vi "Live_Example_XCite_IMAQ.vi"() -> ()   [LabVIEW 2019]
doc: "This example demonstrates the image acquisition with one camera in ring buffer mode together with a live display of the latest images during record. Control of an X-Cite® light source is also possible. After record is stopped, the images can be addressed by index.\nNote that this example will not be fail save, i.e. doesnt react on errors, just handles them forward to the end\n\nUsage:\nSelect your required image count, data format and the camera setup before you start the program.\nOnce started, the camera class will be initialized and images will be recorded and displayed automatically\nYou can stop the images by pressing stop record.\nAfter stopped, the image at the selected index will be read out.\nA search for X-Cite® devices is started, and if found controls are initialized for each channel\nChannels can be switched on and off, and the intensity adjusted while the camera is acquiring images.\nWhen the recording is stopped, all the X-Cite® channels are switched off and controls are disabled.\nTo finish the program click on quit application, this will force an exit of the camera class\nYou can change your required ROI after and also during the record."
uses:
  camera/Camera.lvclass
  pco.sdk/TimingControl/TimingControl.lvlib
  <vilib>/Utility/miscctls.llb/LVOutOfRangeActionTypeDef.ctl
  xcite/Xcite.lvclass
panel:
  in  "type":u16(ring)=65535 items=["XC_120PC"=0, "XC_exacte"=1, "XC_120LED"=2, "XC_110LED"=3, "XC_mini"=4, "XC_XYLIS"=5, "XC_XR210"=6, "XC_LED1"=7, "XC_XT600"=8, "XC_XT900"=9, "Any"=65535]
  in  "Channel9_On":bool caption="735 nm"
  in  "Channel9_Intensity":u32 caption="735 nm" min=5 max=100
  in  "Channel8_On":bool caption="635 nm"
  in  "Channel8_Intensity":u32 caption="635 nm" min=5 max=100
  in  "Channel7_On":bool caption="580 nm"
  in  "Channel7_Intensity":u32 caption="580 nm" min=5 max=100
  in  "Channel6_On":bool caption="555 nm"
  in  "Channel6_Intensity":u32 caption="555 nm" min=5 max=100
  in  "Channel5_On":bool caption="510 nm"
  in  "Channel5_Intensity":u32 caption="510 nm" min=5 max=100
  in  "Channel4_On":bool caption="550 nm"
  in  "Channel4_Intensity":u32 caption="550 nm" min=5 max=100
  in  "Channel3_On":bool caption="475 nm"
  in  "Channel3_Intensity":u32 caption="475 nm" min=5 max=100
  in  "Channel2_On":bool caption="430 nm"
  in  "Channel2_Intensity":u32 caption="430 nm" min=5 max=100
  in  "Channel1_On":bool caption="385 nm"
  in  "Channel1_Intensity":u32 caption="385 nm" min=5 max=100
  out "X-Cite® Model":u16(ring)=65535 items=["XC_120PC"=0, "XC_exacte"=1, "XC_120LED"=2, "XC_110LED"=3, "XC_mini"=4, "XC_XYLIS"=5, "XC_XR210"=6, "XC_LED1"=7, "XC_XT600"=8, "XC_XT900"=9, "Any"=65535]
  in  "Trigger":bool
  in  "data_format":T1(ring)=enum."Mono16"
  out "Image":T2(plugin-control)
  out "rawImage":u16[][](array[numeric])
  in  "Image Index":u32 max=9
  out "Recorded Images":u32
  in  "TriggerMode":T3(ring)
  in  "Quit":bool
  out "Error":errorcluster {"code" format="%x"}
  in  "Stop Record":bool
  out "Recording On":bool
  in  "cropY1":u64=2 min=1 max=1040 step=1
  in  "cropX1":u64=2 min=1 max=1392 step=1
  in  "cropY0":u64=1 min=1 max=1039 step=1
  in  "cropX0":u64=1 min=1 max=1391 step=1
  out "Image Height":u64
  out "Image Width":u64
  in  "dwImgCount":u32=10 caption="Required Number of Images" max=2397
  in  "Exposure Time [s]":dbl=0.010000000000000002 min=1e-06 max=60.0 step=0.001
  # "This example demonstrates the image acquisition with one camera in ring buffer mode together with a live display of the latest images during record. Control of an X-Cite® light source is also possible. After record is stopped, the images can be addressed by index.\nNote that this example will not be fail save, i.e. doesnt react on errors, just handles them forward to the end\n\nUsage:\nSelect your required image count, data format and the camera setup before you start the program.\nOnce started, the camera class will be initialized and images will be recorded and displayed automatically\nYou can stop the images by pressing stop record.\nAfter stopped, the image at the selected index will be read out.\nA search for X-Cite® devices is started, and if found controls are initialized for each channel\nChannels can be switched on and off, and the intensity adjusted while the camera is acquiring images.\nWhen the recording is stopped, all the X-Cite® channels are switched off and controls are disabled.\nTo finish the program click on quit application, this will force an exit of the camera class\nYou can change the cropped region during or after recording."
  # "pco.labview"
  # "Camera Setup"
  # "X-Cite® controls"
  # "Recording Control"
  # "Parameters for image readout"
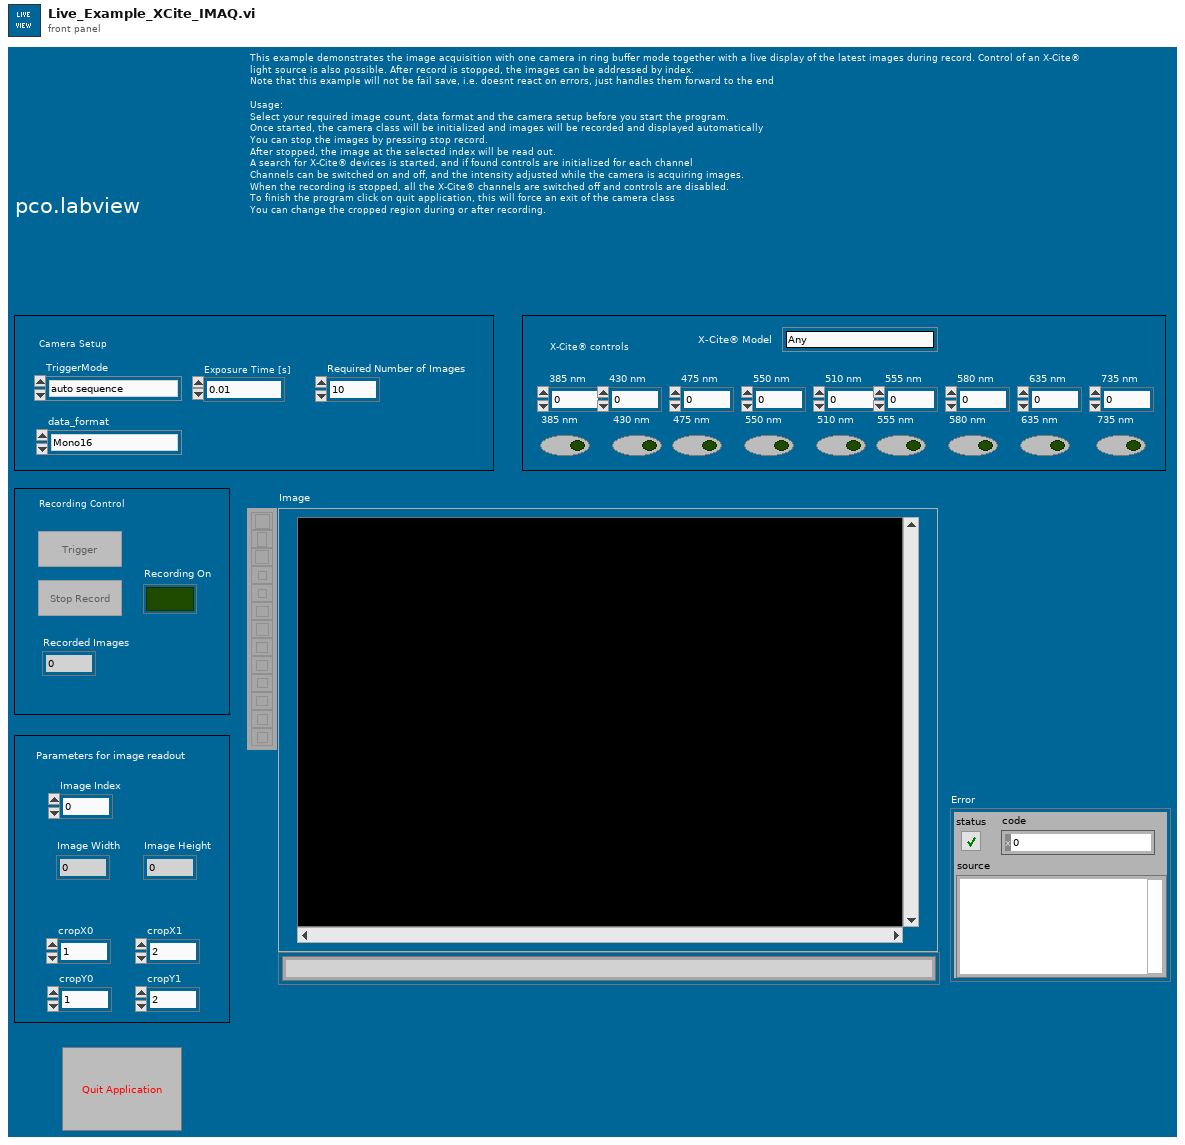
[diagram p1: front panel]
types:
  T1 = enum16{"Undefined", "Mono8", "Mono16", "BGRA8", "RGBA8", "BGRA16", "RGBA16", "CompressedMono8"}
  T2 = typedef "IMAQ Image.ctl" = refnum<image>
  T3 = enum16{"auto sequence", "software trigger", "external exposure start", "external exposure control"}
  T4 = enum8{"Enabled", "Disabled", "Disabled and Grayed Out"}
  T5 = cluster{"serial":u32, "type":u16, "name":string, "wavelenghts_vec":u32[], "exclusivity_vec":u32[], "intensity_max_vec":u32[], "intensity_min_vec":u32[]}
  T6 = enum16{"sequence", "sequence non blocking", "ring buffer", "fifo", "tif", "multitif", "pcoraw", "b16", "dicom", "multidicom", "camram_ring", "camram_segment"}
  T7 = typedef "LVOutOfRangeActionTypeDef.ctl" = cluster{"Out of Range Action Minimum":u8, "Out of Range Action Maximum":u8, "Out of Range Action Increment":u8}
  T8 = cluster{"serial":u32, "type":u16, "sub_type":u16, "interface_type":u16, "bit_resolution":u16, "min_exposure_time_s":dbl, "max_exposure_time_s":dbl, "min_exposure_step_s":dbl, "min_delay_time_s":dbl, "max_delay_time_s":dbl, "min_delay_step_s":dbl, "min_width":u64, "min_height":u64, "max_width":u64, "max_height":u64, "roi_step_horz":u64, "roi_step_vert":u64, "roi_symmetric_horz":bool, "roi_symmetric_vert":bool, "has_timestamp_mode":bool, "has_timestamp_mode_ascii_only":bool, "pixelrate_vec":u32[], "conversion_factor_vec":sgl[], "has_trigger_mode_extexpctrl":bool, "has_acquire_mode":bool, "has_ext_acquire_mode":bool, "has_metadata_mode":bool, "has_ram":bool, "binning_horz_vec":u16[], "binning_vert_vec":u16[], "has_average_binning":bool, "pixel_format_vec":u32[]}
  T9 = typedef "Image Type" = u32
  T10 = cluster{"wSignalNum":u16, "wEnabled":u16, "wType":u16, "wPolarity":u16, "wFilterSetting":u16, "wSelected":u16, "dwParameter":u32[], "dwSignalFunctionality":u32[]}
  T11 = typedef "Camera.lvclass/binning.ctl" = cluster{"vert":u16, "horz":u16, "mode":u16}
  T12 = cluster{"exposure_time_s":dbl, "delay_time_s":dbl, "roi":cluster{"x0":u64, "y0":u64, "x1":u64, "y1":u64}, "timestamp_mode":u16, "pixelrate":u32, "conversion_factor":sgl, "trigger_mode":u16, "acquire_mode":u16, "acquire_sequence_number":u32, "metadata_mode":u16, "noisefilter_mode":u16, "pixel_format":u32, "binning":T11, "auto_exposure":cluster{"region":u16, "min_exposure_s":dbl, "max_exposure_s":dbl}}
  T13 = cluster{"Plane 4 (alpha)":u16, "Plane 1 (Red)":u16, "Plane 2 (Green)":u16, "Plane 3 (Blue)":u16}[][]
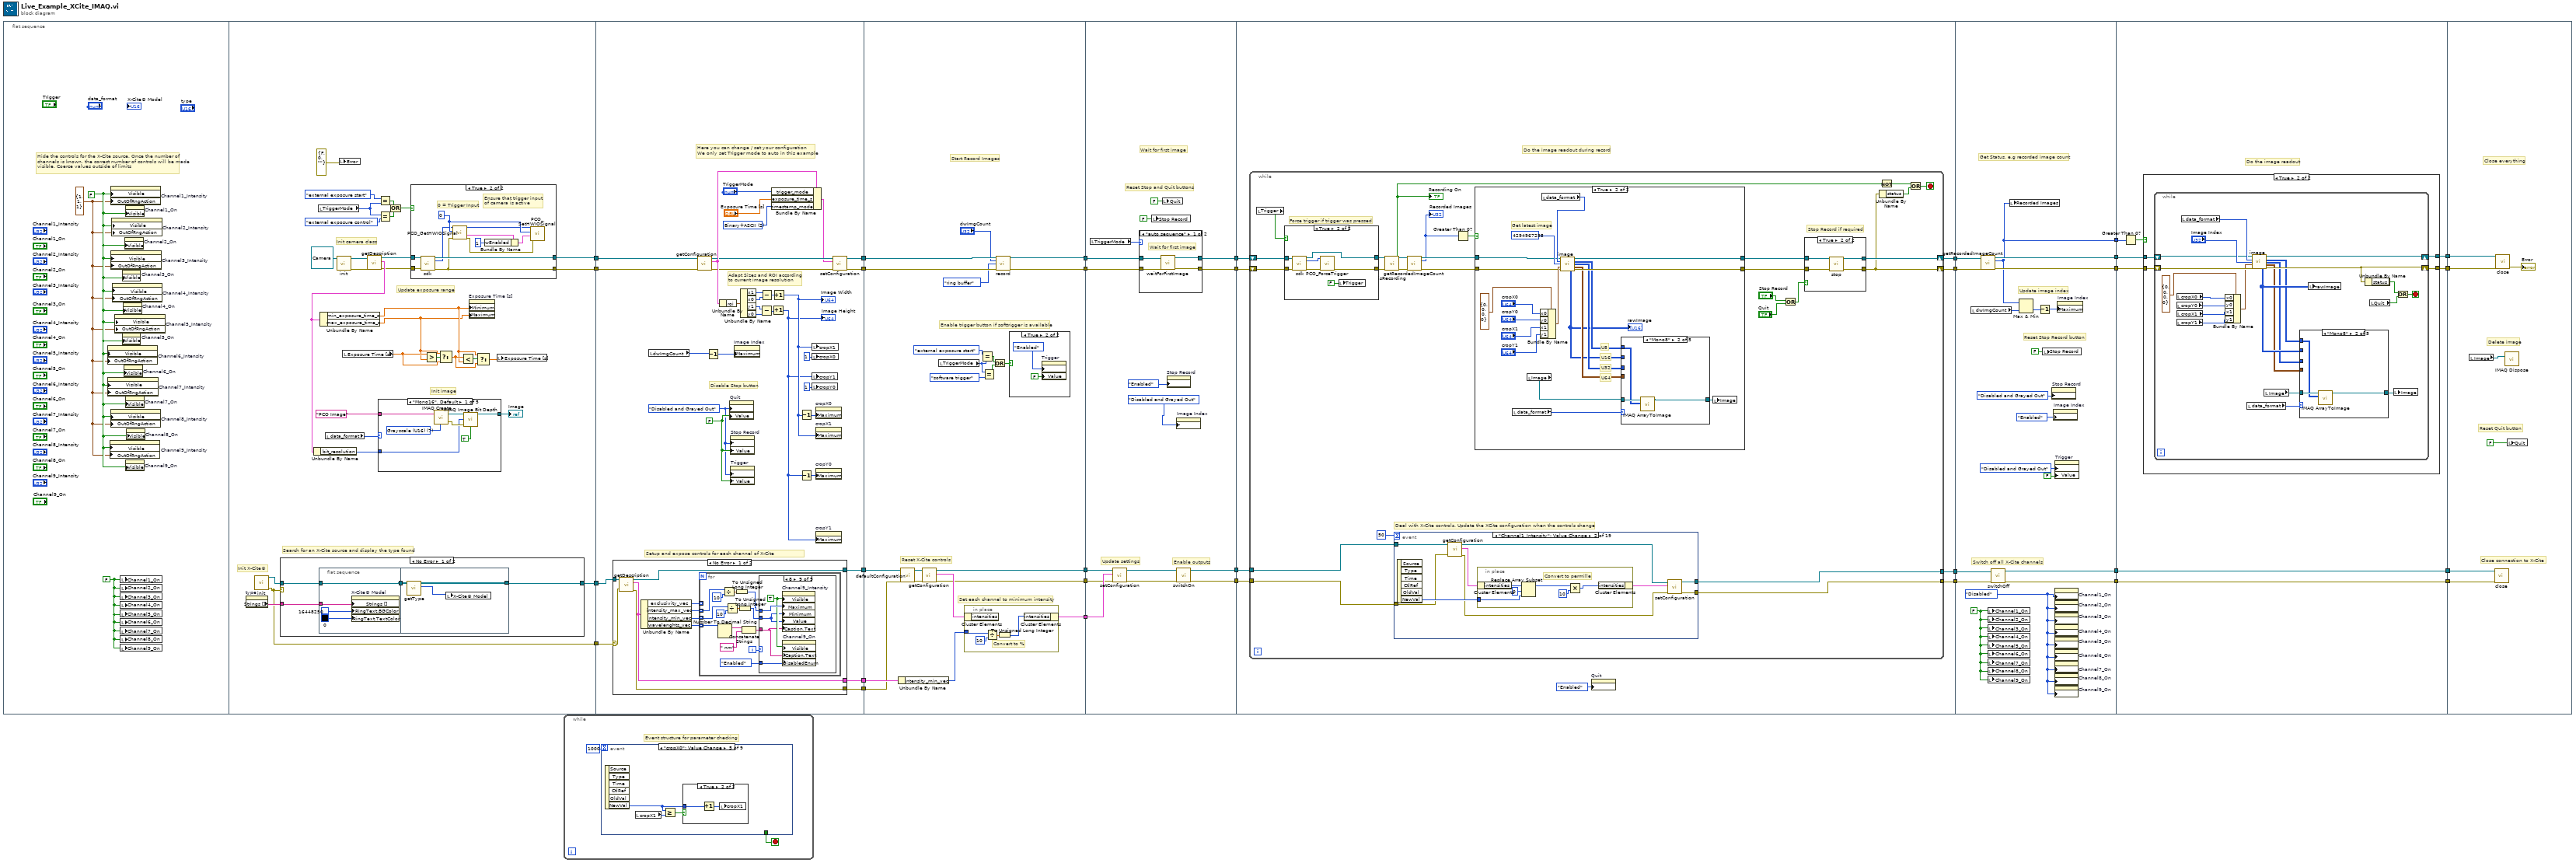
[diagram p0: block diagram]
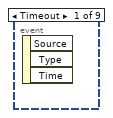
[diagram p2: hidden frame]
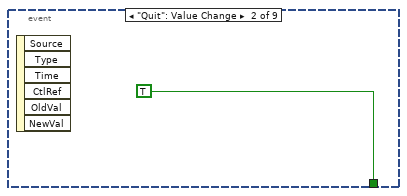
[diagram p3: hidden frame]
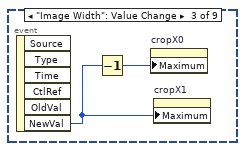
[diagram p4: hidden frame]
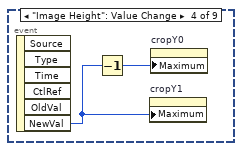
[diagram p5: hidden frame]
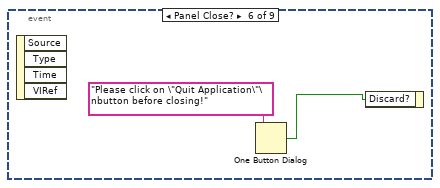
[diagram p7: hidden frame]
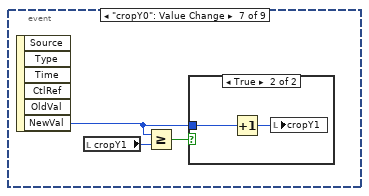
[diagram p8: hidden frame]
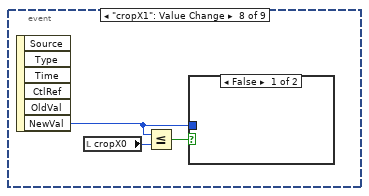
[diagram p10: hidden frame]
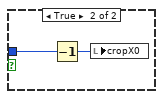
[diagram p11: hidden frame]
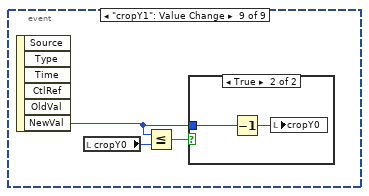
[diagram p12: hidden frame]
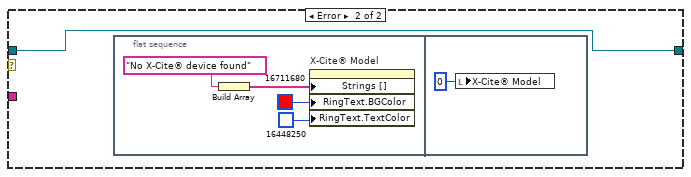
[diagram p14: hidden frame]
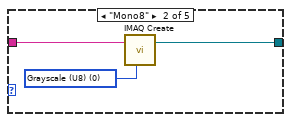
[diagram p16: hidden frame]
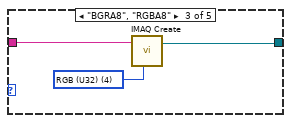
[diagram p17: hidden frame]
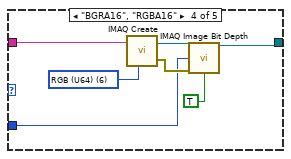
[diagram p18: hidden frame]
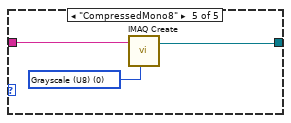
[diagram p19: hidden frame]
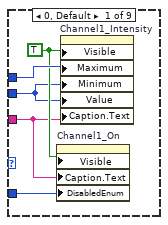
[diagram p20: hidden frame]
diagram:
  n1 = flat-sequence {
    tunnel: [w46] -> w23
    tunnel: [w45] -> w22
    tunnel: [w36] -> w16
    tunnel: [w35] -> w15
    tunnel: [w127] -> w31
    tunnel: [w131] -> w30
    tunnel: w23 -> [w126]
    tunnel: w22 -> [w125]
    tunnel: w16 -> [w122]
    tunnel: w15 -> [w121]
    tunnel: [w120] -> w14
    tunnel: [w119] -> w13
    tunnel: [w118] -> w12
    tunnel: [w233] -> w25
    tunnel: [w234] -> w24
    tunnel: w30 -> [w243]
    tunnel: w31 -> [w242]
    tunnel: w14 -> [w228]
    tunnel: w13 -> [w227]
    tunnel: w12 -> [w226]
    tunnel: [w225] -> w11
    tunnel: [w224] -> w10
    tunnel: [w223] -> w9
    tunnel: w25 -> [w261]
    tunnel: w24 -> [w262]
    tunnel: [w260] -> w29
    tunnel: [w258] -> w18
    tunnel: w11 -> [w254]
    tunnel: w10 -> [w250]
    tunnel: w9 -> [w253]
    tunnel: [w252] -> w8
    tunnel: [w251] -> w7
    tunnel: w29 -> [w280]
    tunnel: [w278] -> w28
    tunnel: [w277] -> w21
    tunnel: w18 -> [w276]
    tunnel: w8 -> [w275]
    tunnel: w7 -> [w274]
    tunnel: [w273] -> w6
    tunnel: [w272] -> w5
    tunnel: w28 -> [w637]
    tunnel: [w635] -> w27
    tunnel: w21 -> [w630]
    tunnel: [w629] -> w20
    tunnel: [w628] -> w17
    tunnel: w6 -> [w625]
    tunnel: w5 -> [w624]
    tunnel: [w623] -> w4
    tunnel: [w622] -> w3
    tunnel: w27 -> [w648]
    tunnel: [w647] -> w26
    tunnel: w20 -> [w646]
    tunnel: [w645] -> w19
    tunnel: w17 -> [w643]
    tunnel: w4 -> [w642]
    tunnel: w3 -> [w641]
    tunnel: [w642] -> w2
    tunnel: [w641] -> w1
    tunnel: w26 -> [w697]
    tunnel: w19 -> [w695]
    tunnel: w2 -> [w693]
    tunnel: w1 -> [w692]
    frame #0 {
      w32 = FALSE ("Channel1_On")
      w33 = T7 {"Out of Range Action Minimum"=1, "Out of Range Action Maximum"=1, "Out of Range Action Increment"=1} ("Response to Value Outside Limits")
      w34 = FALSE
      # "Hide the controls for the X-Cite source. Once the number of channels is known, the correct number of controls will be made visible. Coerce values outside of limits"
      n2 = property on="Channel6_Intensity" class="DigNum (strict)"("Visible"=w34, "OutOfRngAction"=w33) -> ()  [unwired: 2 in, 2 out]
      n3 = property on="Channel7_Intensity" class="DigNum (strict)"("Visible"=w34, "OutOfRngAction"=w33) -> ()  [unwired: 2 in, 2 out]
      n4 = property on="Channel9_Intensity" class="DigNum (strict)"("Visible"=w34, "OutOfRngAction"=w33) -> ()  [unwired: 2 in, 2 out]
      n5 = property on="Channel1_Intensity" class="DigNum (strict)"("Visible"=w34, "OutOfRngAction"=w33) -> ()  [unwired: 2 in, 2 out]
      n6 = property on="Channel8_Intensity" class="DigNum (strict)"("Visible"=w34, "OutOfRngAction"=w33) -> ()  [unwired: 2 in, 2 out]
      n7 = property on="Channel3_Intensity" class="DigNum (strict)"("Visible"=w34, "OutOfRngAction"=w33) -> ()  [unwired: 2 in, 2 out]
      n8 = property on="Channel2_Intensity" class="DigNum (strict)"("Visible"=w34, "OutOfRngAction"=w33) -> ()  [unwired: 2 in, 2 out]
      n9 = property on="Channel4_Intensity" class="DigNum (strict)"("Visible"=w34, "OutOfRngAction"=w33) -> ()  [unwired: 2 in, 2 out]
      n10 = property on="Channel5_Intensity" class="DigNum (strict)"("Visible"=w34, "OutOfRngAction"=w33) -> ()  [unwired: 2 in, 2 out]
      n11 = local write "Channel1_On"(w32) -> ()
      n12 = local write "Channel2_On"(w32) -> ()
      n13 = local write "Channel3_On"(w32) -> ()
      n14 = local write "Channel4_On"(w32) -> ()
      n15 = local write "Channel5_On"(w32) -> ()
      n16 = local write "Channel6_On"(w32) -> ()
      n17 = local write "Channel7_On"(w32) -> ()
      n18 = local write "Channel8_On"(w32) -> ()
      n19 = local write "Channel9_On"(w32) -> ()
      n20 = property on="Channel3_On" class="Bool (strict)"("Visible"=w34) -> ()  [unwired: 2 in, 2 out]
      n21 = property on="Channel5_On" class="Bool (strict)"("Visible"=w34) -> ()  [unwired: 2 in, 2 out]
      n22 = property on="Channel4_On" class="Bool (strict)"("Visible"=w34) -> ()  [unwired: 2 in, 2 out]
      n23 = property on="Channel6_On" class="Bool (strict)"("Visible"=w34) -> ()  [unwired: 2 in, 2 out]
      n24 = property on="Channel2_On" class="Bool (strict)"("Visible"=w34) -> ()  [unwired: 2 in, 2 out]
      n25 = property on="Channel7_On" class="Bool (strict)"("Visible"=w34) -> ()  [unwired: 2 in, 2 out]
      n26 = property on="Channel9_On" class="Bool (strict)"("Visible"=w34) -> ()  [unwired: 2 in, 2 out]
      n27 = property on="Channel1_On" class="Bool (strict)"("Visible"=w34) -> ()  [unwired: 2 in, 2 out]
      n28 = property on="Channel8_On" class="Bool (strict)"("Visible"=w34) -> ()  [unwired: 2 in, 2 out]
    }
    frame #1 {
      # "Search for an X-Cite source and display the type found"
      # "Init X-Cite®"
      # "Init image"
      # "Init camera class"
      # "Update exposure range"
      n29 = property on="type" class="Ring (strict)"() -> ("Strings []"=w37:string[])  [unwired: 2 in, 2 out]
      n30 = call "init.vi"() -> ("error out"=w35:errorcluster, "Xcite out"=w38:refnum<class "Xcite.lvclass">)  [unwired: 10 in]
      n31 = case shown="No Error" w35 {
        tunnel: w38 -> [w66 w76]
        tunnel: [w67 w76] -> w36
        tunnel: w37 -> [w68 _]
        frame No Error {
          n32 = flat-sequence {
            tunnel: w68 -> [w71]
            tunnel: w66 -> [w72]
            tunnel: [w72] -> w65
            tunnel: [w75] -> w67
            tunnel: w65 -> [w74]
            frame #0 {
              n33 = property on="X-Cite® Model" class="Ring (strict)"("Strings []"=w71, "RingText.BGColor"=u32 16448250 ("Ring Text.Colors:BG Color"), "RingText.TextColor"=u32 0 ("Ring Text.Colors:FG Color")) -> ()  [unwired: 2 in, 2 out]
            }
            frame #1 {
              n34 = call "getType.vi"("Xcite in"=w74) -> ("type"=w73:u16, "Xcite out"=w75:refnum<class "Xcite.lvclass">)  [unwired: 8 in, 1 out]
              n35 = local write "X-Cite® Model"(w73) -> ()
            }
          }
        }
        frame Error {
          n36 = flat-sequence {
            frame #0 {
              n37 = Build Array("No X-Cite® device found") -> (w79:string[])
              n38 = property on="X-Cite® Model" class="Ring (strict)"("Strings []"=w79, "RingText.BGColor"=u32 16711680 ("Ring Text.Colors:BG Color"), "RingText.TextColor"=u32 16448250 ("Ring Text.Text Colors:Text Color")) -> ()  [unwired: 2 in, 2 out]
            }
            frame #1 {
              n39 = local write "X-Cite® Model"(0) -> ()
            }
          }
        }
      }
      n40 = local read "TriggerMode"() -> (w40:T3)
      n41 = local read "data_format"() -> (w51:T1)
      n42 = call-dynamic "init.vi"("Camera in"=refnum<class "Camera.lvclass"> refnum) -> ("Camera out"=w54:refnum<class "Camera.lvclass">, "error out"=w55:errorcluster)  [unwired: 8 in]
      n43 = local write "Error"(errorcluster {"status"=FALSE, "code"=0, "source"=""} ("error IO")) -> ()
      n44 = local read "Exposure Time [s]"() -> (w63:dbl)
      n45 = call-dynamic "getDescription.vi"("error in (no error)"=w55, "Camera in"=w54) -> ("error out"=w47:errorcluster, "description"=w50:T8, "Camera out"=w48:refnum<class "Camera.lvclass">)  [unwired: 7 in]
      n46 = Unbundle By Name(w50) -> ("bit_resolution"=w49:u16)
      n47 = Unbundle By Name(w50) -> ("min_exposure_time_s"=w53:dbl, "max_exposure_time_s"=w52:dbl)
      n48 = case shown="\"Mono16\", Default" w51 {
        tunnel: "PCO Image" ("Image Name") -> [w100 w104 w106 w113 w116]
        tunnel: [w96 w102 w105 w110 w115] -> w56
        tunnel: w49 -> [w95 _ _ w108 _]
        frame "Mono16", Default {
          w101 = T9 7 items=["Grayscale (U8)", "Grayscale (I16)", "Grayscale (SGL)", "Complex (CSG)", "RGB (U32)", "HSL (U32)", "RGB (U64)", "Grayscale (U16)"] ("Image Type")
          n49 = call "IMAQ Create"("Image Name"=w100, "Image Type"=w101) -> ("New Image"=w98:T2, "error out"=w97:errorcluster)  [unwired: 3 in]
          n50 = call "IMAQ Image Bit Depth"("Image"=w98, "Bit Depth (0)"=w95, "error in (no error)"=w97, "Get/Set Bit Depth? (Set)"=TRUE) -> ("Image Out"=w96:T2)  [unwired: 9 in, 2 out]
        }
        frame "Mono8" {
          w103 = T9 0 items=["Grayscale (U8)", "Grayscale (I16)", "Grayscale (SGL)", "Complex (CSG)", "RGB (U32)", "HSL (U32)", "RGB (U64)", "Grayscale (U16)"] ("Image Type")
          n51 = call "IMAQ Create"("Image Name"=w104, "Image Type"=w103) -> ("New Image"=w102:T2)  [unwired: 3 in, 1 out]
        }
        frame "BGRA8", "RGBA8" {
          w107 = T9 4 items=["Grayscale (U8)", "Grayscale (I16)", "Grayscale (SGL)", "Complex (CSG)", "RGB (U32)", "HSL (U32)", "RGB (U64)", "Grayscale (U16)"] ("Image Type")
          n52 = call "IMAQ Create"("Image Name"=w106, "Image Type"=w107) -> ("New Image"=w105:T2)  [unwired: 3 in, 1 out]
        }
        frame "BGRA16", "RGBA16" {
          w114 = T9 6 items=["Grayscale (U8)", "Grayscale (I16)", "Grayscale (SGL)", "Complex (CSG)", "RGB (U32)", "HSL (U32)", "RGB (U64)", "Grayscale (U16)"] ("Image Type")
          n53 = call "IMAQ Create"("Image Name"=w113, "Image Type"=w114) -> ("New Image"=w111:T2, "error out"=w109:errorcluster)  [unwired: 3 in]
          n54 = call "IMAQ Image Bit Depth"("Image"=w111, "Bit Depth (0)"=w108, "error in (no error)"=w109, "Get/Set Bit Depth? (Set)"=TRUE) -> ("Image Out"=w110:T2)  [unwired: 9 in, 2 out]
        }
        frame "CompressedMono8" {
          w117 = T9 0 items=["Grayscale (U8)", "Grayscale (I16)", "Grayscale (SGL)", "Complex (CSG)", "RGB (U32)", "HSL (U32)", "RGB (U64)", "Grayscale (U16)"] ("Image Type")
          n55 = call "IMAQ Create"("Image Name"=w116, "Image Type"=w117) -> ("New Image"=w115:T2)  [unwired: 3 in, 1 out]
        }
      }
      "Image" <- w56
      n56 = Equal?(x=T3."external exposure start" ("TriggerMode"), y=w40) -> (x = y?=w43:bool)
      n57 = Equal?(x=w40, y=T3."external exposure control" ("TriggerMode")) -> (x = y?=w42:bool)
      n58 = Or(x=w43, y=w42) -> (x .or. y?=w41:bool)
      n59 = case shown="True" w41 {
        tunnel: w48 -> [w83 w88]
        tunnel: w47 -> [w82 w87]
        tunnel: [w83 w86] -> w46
        tunnel: [w82 w84] -> w45
        frame False {
        }
        frame True {
          w92 = u16 0 ("wSignalNum")
          # "0 = Trigger Input"
          # "Ensure that trigger input\nof camera is active"
          n60 = call-dynamic "sdk.vi"("Camera in"=w88, "error in (no error)"=w87) -> ("Camera out"=w86:refnum<class "Camera.lvclass">, "sdk"=w85:u64, "error out"=w84:errorcluster)  [unwired: 11 in]
          n61 = call "PCO_GetHWIOSignal.vi"("error in (no error)"=w84, "wSignalNum"=w92, "ph"=w85) -> ("error out"=w90:errorcluster, "strSignal"=w94:T10, "ph out"=w89:u64)  [unwired: 5 in, 1 out]
          n62 = Bundle By Name(cluster=w94, "wEnabled"=u16 1) -> (w91:T10)
          n63 = call "PCO_SetHWIOSignal.vi"("error in (no error)"=w90, "strSignal"=w91, "wSignalNum"=w92, "ph"=w89) -> ()  [unwired: 5 in, 3 out]
        }
      }
      n64 = Greater?(x=w63, y=w52) -> (0:w64:bool)
      n65 = Select(t=w52, s=w64, f=w63) -> (s? t:f=w61:dbl)
      n66 = Less?(x=w61, y=w53) -> (x < y?=w62:bool)
      n67 = property on="Exposure Time [s]" class="DigNum (strict)"("Minimum"=w53, "Maximum"=w52) -> ()  [unwired: 2 in, 2 out]
      n68 = Select(t=w53, s=w62, f=w61) -> (s? t:f=w60:dbl)
      n69 = local write "Exposure Time [s]"(w60) -> ()
    }
    frame #2 {
      w137 = u16 2 items=["OFF", "Binary", "Binary+ASCII", "ASCII"] ("wTimeStampMode")
      w124 = FALSE ("Stop")
      w123 = T4."Disabled and Grayed Out" ("Disabled")
      # "Setup and expose controls for each channel of X-Cite"
      # "Disable Stop button"
      # "Adapt Sizes and ROI according\nto current image resolution"
      # "Here you can change / set your configuration\nWe only set Trigger mode to auto in this example"
      n70 = case shown="No Error" w121 {
        selector: w121 -> [w152 w219]
        tunnel: w122 -> [w159 w221]
        tunnel: [w158 w221] -> w120
        tunnel: [w153 T5 {"serial"=0, "type"=0, "name"="", "wavelenghts_vec"=[], "exclusivity_vec"=[], "intensity_max_vec"=[], "intensity_min_vec"=[]} ("XCITE_Description")] -> w119
        tunnel: [w151 w219] -> w118
        frame No Error {
          n71 = call "getDescription.vi"("error in (no error)"=w152, "Xcite in"=w159) -> ("error out"=w151:errorcluster, "description"=w153:T5, "Xcite out"=w158:refnum<class "Xcite.lvclass">)  [unwired: 7 in]
          n72 = Unbundle By Name(w153) -> ("exclusivity_vec"=w157:u32[], "intensity_max_vec"=w156:u32[], "intensity_min_vec"=w155:u32[], "wavelenghts_vec"=w154:u32[])
          n73 = for {
            tunnel: w157 -> [_] mode=indexing
            tunnel: w156 -> [w167] mode=indexing
            tunnel: w155 -> [w162] mode=indexing
            tunnel: w154 -> [w172] mode=indexing
            i -> [w173]
            n74 = Number To Decimal String(number=w172) -> (decimal integer string=w171:string)  [unwired: 1 in]
            n75 = Divide(x=w167, y=u32 10) -> (x/y=w165:dbl)
            n76 = Divide(x=w162, y=u32 10) -> (x/y=w163:dbl)
            n77 = To Unsigned Long Integer(number=w165) -> (unsigned 32bit integer=w160:u32)
            n78 = To Unsigned Long Integer(number=w163) -> (unsigned 32bit integer=w161:u32)
            n79 = Concatenate Strings(w171, " nm") -> (w169:string)
            n80 = case shown="8" w173 {
              tunnel: w169 -> [w175 w180 w185 w191 w196 w201 w205 w211 w216]
              tunnel: w160 -> [w178 w183 w188 w193 w198 w203 w208 w213 w218]
              tunnel: w161 -> [w176 w181 w186 w190 w195 w200 w206 w210 w215]
              tunnel: T4."Enabled" ("Disabled") -> [w174 w179 w184 w189 w194 w199 w204 w209 w214]
              frame 0, Default {
                w177 = TRUE ("Visible")
                n81 = property on="Channel1_On" class="Bool (strict)"("Visible"=w177, "Caption.Text"=w175, "DisabledEnum"=w174) -> ()  [unwired: 2 in, 2 out]
                n82 = property on="Channel1_Intensity" class="DigNum (strict)"("Visible"=w177, "Maximum"=w178, "Minimum"=w176, "Value"=w176, "Caption.Text"=w175) -> ()  [unwired: 2 in, 2 out]
              }
              frame 1 {
                w182 = TRUE ("Visible")
                n83 = property on="Channel2_Intensity" class="DigNum (strict)"("Visible"=w182, "Maximum"=w183, "Minimum"=w181, "Value"=w181, "Caption.Text"=w180) -> ()  [unwired: 2 in, 2 out]
                n84 = property on="Channel2_On" class="Bool (strict)"("Visible"=w182, "Caption.Text"=w180, "DisabledEnum"=w179) -> ()  [unwired: 2 in, 2 out]
              }
              frame 2 {
                w187 = TRUE ("Visible")
                n85 = property on="Channel3_On" class="Bool (strict)"("Visible"=w187, "Caption.Text"=w185, "DisabledEnum"=w184) -> ()  [unwired: 2 in, 2 out]
                n86 = property on="Channel3_Intensity" class="DigNum (strict)"("Visible"=w187, "Maximum"=w188, "Minimum"=w186, "Value"=w186, "Caption.Text"=w185) -> ()  [unwired: 2 in, 2 out]
              }
              frame 3 {
                w192 = TRUE ("Visible")
                n87 = property on="Channel4_Intensity" class="DigNum (strict)"("Visible"=w192, "Maximum"=w193, "Minimum"=w190, "Value"=w190, "Caption.Text"=w191) -> ()  [unwired: 2 in, 2 out]
                n88 = property on="Channel4_On" class="Bool (strict)"("Visible"=w192, "Caption.Text"=w191, "DisabledEnum"=w189) -> ()  [unwired: 2 in, 2 out]
              }
              frame 4 {
                w197 = TRUE ("Visible")
                n89 = property on="Channel5_Intensity" class="DigNum (strict)"("Visible"=w197, "Maximum"=w198, "Minimum"=w195, "Value"=w195, "Caption.Text"=w196) -> ()  [unwired: 2 in, 2 out]
                n90 = property on="Channel5_On" class="Bool (strict)"("Visible"=w197, "Caption.Text"=w196, "DisabledEnum"=w194) -> ()  [unwired: 2 in, 2 out]
              }
              frame 5 {
                w202 = TRUE ("Visible")
                n91 = property on="Channel6_Intensity" class="DigNum (strict)"("Visible"=w202, "Maximum"=w203, "Minimum"=w200, "Value"=w200, "Caption.Text"=w201) -> ()  [unwired: 2 in, 2 out]
                n92 = property on="Channel6_On" class="Bool (strict)"("Visible"=w202, "Caption.Text"=w201, "DisabledEnum"=w199) -> ()  [unwired: 2 in, 2 out]
              }
              frame 6 {
                w207 = TRUE ("Visible")
                n93 = property on="Channel7_Intensity" class="DigNum (strict)"("Visible"=w207, "Maximum"=w208, "Minimum"=w206, "Value"=w206, "Caption.Text"=w205) -> ()  [unwired: 2 in, 2 out]
                n94 = property on="Channel7_On" class="Bool (strict)"("Visible"=w207, "Caption.Text"=w205, "DisabledEnum"=w204) -> ()  [unwired: 2 in, 2 out]
              }
              frame 7 {
                w212 = TRUE ("Visible")
                n95 = property on="Channel8_Intensity" class="DigNum (strict)"("Visible"=w212, "Maximum"=w213, "Minimum"=w210, "Value"=w210, "Caption.Text"=w211) -> ()  [unwired: 2 in, 2 out]
                n96 = property on="Channel8_On" class="Bool (strict)"("Visible"=w212, "Caption.Text"=w211, "DisabledEnum"=w209) -> ()  [unwired: 2 in, 2 out]
              }
              frame 8 {
                w217 = TRUE ("Visible")
                n97 = property on="Channel9_Intensity" class="DigNum (strict)"("Visible"=w217, "Maximum"=w218, "Minimum"=w215, "Value"=w215, "Caption.Text"=w216) -> ()  [unwired: 2 in, 2 out]
                n98 = property on="Channel9_On" class="Bool (strict)"("Visible"=w217, "Caption.Text"=w216, "DisabledEnum"=w214) -> ()  [unwired: 2 in, 2 out]
              }
            }
          }
        }
        frame Error {
        }
      }
      n99 = local read "dwImgCount"() -> (w138:u32)
      n100 = call-dynamic "getConfiguration.vi"("error in (no error)"=w125, "Camera in"=w126) -> ("error out"=w132:errorcluster, "configuration"=w143:T12, "Camera out"=w134:refnum<class "Camera.lvclass">)  [unwired: 7 in]
      n101 = Decrement(x=w138) -> (x-1=w128:u32)
      n102 = Unbundle By Name(w143) -> ("roi"=w144:cluster{"x0":u64, "y0":u64, "x1":u64, "y1":u64})
      n103 = property on="Quit" class="Bool (strict)"("DisabledEnum"=w123, "Value"=w124) -> ()  [unwired: 2 in, 2 out]
      n104 = property on="Stop Record" class="Bool (strict)"("DisabledEnum"=w123, "Value"=w124) -> ()  [unwired: 2 in, 2 out]
      n105 = property on="Trigger" class="Bool (strict)"("DisabledEnum"=w123, "Value"=w124) -> ()  [unwired: 2 in, 2 out]
      n106 = property on="Image Index" class="DigNum (strict)"("Maximum"=w128) -> ()  [unwired: 2 in, 2 out]
      n107 = Unbundle By Name(w144) -> ("x1"=w146:u64, "x0"=w145:u64, "y1"=w148:u64, "y0"=w147:u64)
      n108 = Subtract(x=w148, y=w147) -> (x-y=w150:u64)
      n109 = Subtract(x=w146, y=w145) -> (x-y=w149:u64)
      n110 = Bundle By Name(cluster=w143, "trigger_mode"="TriggerMode", "exposure_time_s"="Exposure Time [s]", "timestamp_mode"=w137) -> (w133:T12)
      n111 = Increment(x=w150) -> (x+1=w129:u64)
      "Image Height" <- w129
      n112 = Increment(x=w149) -> (x+1=w130:u64)
      "Image Width" <- w130
      n113 = Decrement(x=w130) -> (x-1=w141:u64)
      n114 = Decrement(x=w129) -> (x-1=w142:u64)
      n115 = local write "cropX1"(w130) -> ()
      n116 = local write "cropX0"(u64 1 ("roiY0")) -> ()
      n117 = local write "cropY1"(w129) -> ()
      n118 = local write "cropY0"(u64 1 ("roiY0")) -> ()
      n119 = property on="cropX0" class="DigNum (strict)"("Maximum"=w141) -> ()  [unwired: 2 in, 2 out]
      n120 = property on="cropX1" class="DigNum (strict)"("Maximum"=w130) -> ()  [unwired: 2 in, 2 out]
      n121 = property on="cropY0" class="DigNum (strict)"("Maximum"=w142) -> ()  [unwired: 2 in, 2 out]
      n122 = property on="cropY1" class="DigNum (strict)"("Maximum"=w129) -> ()  [unwired: 2 in, 2 out]
      n123 = call-dynamic "setConfiguration.vi"("error in (no error)"=w132, "configuration"=w133, "Camera in"=w134) -> ("error out"=w131:errorcluster, "Camera out"=w127:refnum<class "Camera.lvclass">)  [unwired: 7 in]
    }
    frame #3 {
      # "Set each channel to minimum intensity"
      # "Reset X-Cite controls"
      # "Enable trigger button if softtrigger is available"
      # "Start Record Images"
      n124 = Unbundle By Name(w227) -> ("intensity_min_vec"=w229:u32[])
      n125 = call "defaultConfiguration.vi"("error in (no error)"=w226, "Xcite in"=w228) -> ("error out"=w231:errorcluster, "Xcite out"=w232:refnum<class "Xcite.lvclass">)  [unwired: 8 in]
      n126 = call "getConfiguration.vi"("error in (no error)"=w231, "Xcite in"=w232) -> ("error out"=w224:errorcluster, "configuration"=w230:cluster{"intensities":u32[], "on_states":u8[]}, "Xcite out"=w225:refnum<class "Xcite.lvclass">)  [unwired: 7 in]
      n127 = local read "TriggerMode"() -> (w239:T3)
      n128 = in-place {
        in-place-border: w229 -> [w245]
        # "Convert to %"
        n129 = in-place-cluster #1(w230) -> ()  [unwired: 1 out]
        n130 = Divide(x=w245, y=u32 10) -> (x/y=w246:dbl[])
        n131 = To Unsigned Long Integer(number=w246) -> (unsigned 32bit integer=w244:u32[])
        n132 = in-place-cluster #1("intensities"=w244) -> (w223:cluster{"intensities":u32[], "on_states":u8[]})
      }
      n133 = Equal?(x=T3."external exposure start" ("TriggerMode"), y=w239) -> (x = y?=w236:bool)
      n134 = Equal?(x=w239, y=T3."software trigger" ("TriggerMode")) -> (x = y?=w235:bool)
      n135 = Or(x=w236, y=w235) -> (x .or. y?=w237:bool)
      n136 = call-dynamic "record.vi"("Camera in"=w242, "num_images"="dwImgCount", "record_mode"=T6."ring buffer", "error in (no error)"=w243) -> ("Camera out"=w234:refnum<class "Camera.lvclass">, "error out"=w233:errorcluster)  [unwired: 10 in]
      n137 = case shown="True" w237 {
        frame False {
        }
        frame True {
          n138 = property on="Trigger" class="Bool (strict)"("DisabledEnum"=T4."Enabled" ("Disabled"), "Value"=FALSE ("Trigger")) -> ()  [unwired: 2 in, 2 out]
        }
      }
    }
    frame #4 {
      # "Enable outputs"
      # "Update settings"
      # "Wait for first image"
      # "Reset Stop and Quit buttons"
      n139 = local read "TriggerMode"() -> (w257:T3)
      n140 = call "setConfiguration.vi"("error in (no error)"=w250, "configuration"=w253, "Xcite in"=w254) -> ("error out"=w255:errorcluster, "Xcite out"=w256:refnum<class "Xcite.lvclass">)  [unwired: 7 in]
      n141 = case shown="\"auto sequence\"" w257 {
        tunnel: w262 -> [w269 w271]
        tunnel: w261 -> [w268 w270]
        tunnel: [w267 w270] -> w260
        tunnel: [w266 w271] -> w258
        frame "auto sequence" {
          # "Wait for first image"
          n142 = call-dynamic "waitForFirstImage.vi"("error in (no error)"=w268, "Camera in"=w269) -> ("error out"=w267:errorcluster, "Camera out"=w266:refnum<class "Camera.lvclass">)  [unwired: 8 in]
        }
        frame Default {
        }
      }
      n143 = local write "Stop Record"(FALSE ("Stop Record")) -> ()
      n144 = local write "Quit"(FALSE ("Stop")) -> ()
      n145 = property on="Stop Record" class="Bool (strict)"("DisabledEnum"=T4."Enabled" ("Disabled")) -> ()  [unwired: 2 in, 2 out]
      n146 = property on="Image Index" class="DigNum (strict)"("DisabledEnum"=T4."Disabled and Grayed Out" ("Disabled")) -> ()  [unwired: 2 in, 2 out]
      n147 = call "switchOn.vi"("error in (no error)"=w255, "Xcite in"=w256) -> ("error out"=w251:errorcluster, "Xcite out"=w252:refnum<class "Xcite.lvclass">)  [unwired: 8 in]
    }
    frame #5 {
      # "Do the image readout during record"
      n148 = while {
        shift-right: [w288] -> w278
        shift-left: w280 -> [w292]
        shift-right: [w289] -> w277
        shift-left: w276 -> [w293]
        tunnel: w275 -> [w284]
        tunnel: w274 -> [w283]
        tunnel: [w282] -> w273
        tunnel: [w281] -> w272
        stop <- w304 stop-if-true
        # "Deal with X-Cite controls. Update the XCite configuration when the controls change"
        # "Force trigger if trigger was pressed"
        # "Stop Record if required"
        n149 = local read "Trigger"() -> (w294:bool)
        n150 = case shown="True" w294 {
          tunnel: w293 -> [w608 w613]
          tunnel: w292 -> [w607 w612]
          tunnel: [w608 w611] -> w291
          tunnel: [w607 w610] -> w290
          frame False {
          }
          frame True {
            n151 = call-dynamic "sdk.vi"("Camera in"=w613, "error in (no error)"=w612) -> ("Camera out"=w611:refnum<class "Camera.lvclass">, "sdk"=w614:u64, "error out"=w615:errorcluster)  [unwired: 11 in]
            n152 = call "PCO_ForceTrigger.vi"("error in (no error)"=w615, "ph"=w614) -> ("error out"=w610:errorcluster)  [unwired: 6 in, 3 out]
            n153 = local write "Trigger"(FALSE ("Trigger")) -> ()
          }
        }
        n154 = call-dynamic "isRecording.vi"("Camera in"=w291, "error in (no error)"=w290) -> ("Camera out"=w299:refnum<class "Camera.lvclass">, "recording"=w302:bool, "error out"=w298:errorcluster)  [unwired: 11 in]
        "Recording On" <- w302
        n155 = event shown="[1] \"Channel1_Intensity\": Value Change" {
          selector: _ -> [_ _ _ _ _ _ _ _ _ _ _ _ _ _ _ _ _ _ _]
          dyn-events: _ -> [_ _ _ _ _ _ _ _ _ _ _ _ _ _ _ _ _ _ _]
          timeout: 50 -> [_ _ _ _ _ _ _ _ _ _ _ _ _ _ _ _ _ _ _]
          tunnel: w284 -> [w308 w316 w331 w346 w361 w376 w391 w406 w421 w436 w452 w466 w480 w494 w508 w522 w536 w550 w564]
          tunnel: [w309 w315 w330 w345 w360 w375 w390 w405 w420 w435 w451 w465 w479 w493 w507 w521 w535 w549 w563] -> w281
          tunnel: w283 -> [w309 w311 w326 w341 w356 w371 w386 w401 w416 w431 w446 w460 w474 w488 w502 w516 w530 w544 w558]
          tunnel: [w308 w314 w329 w344 w359 w374 w389 w404 w419 w434 w450 w464 w478 w492 w506 w520 w534 w548 w562] -> w282
          event Timeout {
            n156 = event-data() -> ()  [unwired: 1 in, 3 out]
          }
          event "Channel1_Intensity": Value Change {
            n157 = event-data() -> ("NewVal"=w318:u32)  [unwired: 1 in, 5 out]
            n158 = call "getConfiguration.vi"("error in (no error)"=w311, "Xcite in"=w316) -> ("error out"=w310:errorcluster, "configuration"=w312:cluster{"intensities":u32[], "on_states":u8[]}, "Xcite out"=w313:refnum<class "Xcite.lvclass">)  [unwired: 7 in]
            n159 = in-place {
              in-place-border: w318 -> [w322]
              # "Convert to permille"
              n160 = in-place-cluster #2(w312) -> ("intensities"=w324:u32[])
              n161 = Replace Array Subset(array=w324, new element=w322, index=0) -> (w320:u32[])
              n162 = Multiply(x=w320, y=u32 10) -> (x*y=w319:u32[])
              n163 = in-place-cluster #2("intensities"=w319) -> (w317:cluster{"intensities":u32[], "on_states":u8[]})
            }
            n164 = call "setConfiguration.vi"("error in (no error)"=w310, "configuration"=w317, "Xcite in"=w313) -> ("error out"=w315:errorcluster, "Xcite out"=w314:refnum<class "Xcite.lvclass">)  [unwired: 7 in]
          }
          event "Channel2_Intensity": Value Change {
            n165 = event-data() -> ("NewVal"=w333:u32)  [unwired: 1 in, 5 out]
            n166 = call "getConfiguration.vi"("error in (no error)"=w326, "Xcite in"=w331) -> ("error out"=w325:errorcluster, "configuration"=w327:cluster{"intensities":u32[], "on_states":u8[]}, "Xcite out"=w328:refnum<class "Xcite.lvclass">)  [unwired: 7 in]
            n167 = in-place {
              in-place-border: w333 -> [w337]
              # "Convert to permille"
              n168 = in-place-cluster #3(w327) -> ("intensities"=w339:u32[])
              n169 = Replace Array Subset(array=w339, new element=w337, index=1) -> (w335:u32[])
              n170 = Multiply(x=w335, y=u32 10) -> (x*y=w334:u32[])
              n171 = in-place-cluster #3("intensities"=w334) -> (w332:cluster{"intensities":u32[], "on_states":u8[]})
            }
            n172 = call "setConfiguration.vi"("error in (no error)"=w325, "configuration"=w332, "Xcite in"=w328) -> ("error out"=w330:errorcluster, "Xcite out"=w329:refnum<class "Xcite.lvclass">)  [unwired: 7 in]
          }
          event "Channel3_Intensity": Value Change {
            n173 = event-data() -> ("NewVal"=w348:u32)  [unwired: 1 in, 5 out]
            n174 = call "getConfiguration.vi"("error in (no error)"=w341, "Xcite in"=w346) -> ("error out"=w340:errorcluster, "configuration"=w342:cluster{"intensities":u32[], "on_states":u8[]}, "Xcite out"=w343:refnum<class "Xcite.lvclass">)  [unwired: 7 in]
            n175 = in-place {
              in-place-border: w348 -> [w352]
              # "Convert to permille"
              n176 = in-place-cluster #4(w342) -> ("intensities"=w354:u32[])
              n177 = Replace Array Subset(array=w354, new element=w352, index=2) -> (w350:u32[])
              n178 = Multiply(x=w350, y=u32 10) -> (x*y=w349:u32[])
              n179 = in-place-cluster #4("intensities"=w349) -> (w347:cluster{"intensities":u32[], "on_states":u8[]})
            }
            n180 = call "setConfiguration.vi"("error in (no error)"=w340, "configuration"=w347, "Xcite in"=w343) -> ("error out"=w345:errorcluster, "Xcite out"=w344:refnum<class "Xcite.lvclass">)  [unwired: 7 in]
          }
          event "Channel4_Intensity": Value Change {
            n181 = event-data() -> ("NewVal"=w363:u32)  [unwired: 1 in, 5 out]
            n182 = call "getConfiguration.vi"("error in (no error)"=w356, "Xcite in"=w361) -> ("error out"=w355:errorcluster, "configuration"=w357:cluster{"intensities":u32[], "on_states":u8[]}, "Xcite out"=w358:refnum<class "Xcite.lvclass">)  [unwired: 7 in]
            n183 = in-place {
              in-place-border: w363 -> [w367]
              # "Convert to permille"
              n184 = in-place-cluster #5(w357) -> ("intensities"=w369:u32[])
              n185 = Replace Array Subset(array=w369, new element=w367, index=3) -> (w365:u32[])
              n186 = Multiply(x=w365, y=u32 10) -> (x*y=w364:u32[])
              n187 = in-place-cluster #5("intensities"=w364) -> (w362:cluster{"intensities":u32[], "on_states":u8[]})
            }
            n188 = call "setConfiguration.vi"("error in (no error)"=w355, "configuration"=w362, "Xcite in"=w358) -> ("error out"=w360:errorcluster, "Xcite out"=w359:refnum<class "Xcite.lvclass">)  [unwired: 7 in]
          }
          event "Channel5_Intensity": Value Change {
            n189 = event-data() -> ("NewVal"=w378:u32)  [unwired: 1 in, 5 out]
            n190 = call "getConfiguration.vi"("error in (no error)"=w371, "Xcite in"=w376) -> ("error out"=w370:errorcluster, "configuration"=w372:cluster{"intensities":u32[], "on_states":u8[]}, "Xcite out"=w373:refnum<class "Xcite.lvclass">)  [unwired: 7 in]
            n191 = in-place {
              in-place-border: w378 -> [w382]
              # "Convert to permille"
              n192 = in-place-cluster #6(w372) -> ("intensities"=w384:u32[])
              n193 = Replace Array Subset(array=w384, new element=w382, index=4) -> (w380:u32[])
              n194 = Multiply(x=w380, y=u32 10) -> (x*y=w379:u32[])
              n195 = in-place-cluster #6("intensities"=w379) -> (w377:cluster{"intensities":u32[], "on_states":u8[]})
            }
            n196 = call "setConfiguration.vi"("error in (no error)"=w370, "configuration"=w377, "Xcite in"=w373) -> ("error out"=w375:errorcluster, "Xcite out"=w374:refnum<class "Xcite.lvclass">)  [unwired: 7 in]
          }
          event "Channel6_Intensity": Value Change {
            n197 = event-data() -> ("NewVal"=w393:u32)  [unwired: 1 in, 5 out]
            n198 = call "getConfiguration.vi"("error in (no error)"=w386, "Xcite in"=w391) -> ("error out"=w385:errorcluster, "configuration"=w387:cluster{"intensities":u32[], "on_states":u8[]}, "Xcite out"=w388:refnum<class "Xcite.lvclass">)  [unwired: 7 in]
            n199 = in-place {
              in-place-border: w393 -> [w397]
              # "Convert to permille"
              n200 = in-place-cluster #7(w387) -> ("intensities"=w399:u32[])
              n201 = Replace Array Subset(array=w399, new element=w397, index=5) -> (w395:u32[])
              n202 = Multiply(x=w395, y=u32 10) -> (x*y=w394:u32[])
              n203 = in-place-cluster #7("intensities"=w394) -> (w392:cluster{"intensities":u32[], "on_states":u8[]})
            }
            n204 = call "setConfiguration.vi"("error in (no error)"=w385, "configuration"=w392, "Xcite in"=w388) -> ("error out"=w390:errorcluster, "Xcite out"=w389:refnum<class "Xcite.lvclass">)  [unwired: 7 in]
          }
          event "Channel7_Intensity": Value Change {
            n205 = event-data() -> ("NewVal"=w408:u32)  [unwired: 1 in, 5 out]
            n206 = call "getConfiguration.vi"("error in (no error)"=w401, "Xcite in"=w406) -> ("error out"=w400:errorcluster, "configuration"=w402:cluster{"intensities":u32[], "on_states":u8[]}, "Xcite out"=w403:refnum<class "Xcite.lvclass">)  [unwired: 7 in]
            n207 = in-place {
              in-place-border: w408 -> [w412]
              # "Convert to permille"
              n208 = in-place-cluster #8(w402) -> ("intensities"=w414:u32[])
              n209 = Replace Array Subset(array=w414, new element=w412, index=6) -> (w410:u32[])
              n210 = Multiply(x=w410, y=u32 10) -> (x*y=w409:u32[])
              n211 = in-place-cluster #8("intensities"=w409) -> (w407:cluster{"intensities":u32[], "on_states":u8[]})
            }
            n212 = call "setConfiguration.vi"("error in (no error)"=w400, "configuration"=w407, "Xcite in"=w403) -> ("error out"=w405:errorcluster, "Xcite out"=w404:refnum<class "Xcite.lvclass">)  [unwired: 7 in]
          }
          event "Channel8_Intensity": Value Change {
            n213 = event-data() -> ("NewVal"=w423:u32)  [unwired: 1 in, 5 out]
            n214 = call "getConfiguration.vi"("error in (no error)"=w416, "Xcite in"=w421) -> ("error out"=w415:errorcluster, "configuration"=w417:cluster{"intensities":u32[], "on_states":u8[]}, "Xcite out"=w418:refnum<class "Xcite.lvclass">)  [unwired: 7 in]
            n215 = in-place {
              in-place-border: w423 -> [w427]
              # "Convert to permille"
              n216 = in-place-cluster #9(w417) -> ("intensities"=w429:u32[])
              n217 = Replace Array Subset(array=w429, new element=w427, index=7) -> (w425:u32[])
              n218 = Multiply(x=w425, y=u32 10) -> (x*y=w424:u32[])
              n219 = in-place-cluster #9("intensities"=w424) -> (w422:cluster{"intensities":u32[], "on_states":u8[]})
            }
            n220 = call "setConfiguration.vi"("error in (no error)"=w415, "configuration"=w422, "Xcite in"=w418) -> ("error out"=w420:errorcluster, "Xcite out"=w419:refnum<class "Xcite.lvclass">)  [unwired: 7 in]
          }
          event "Channel9_Intensity": Value Change {
            n221 = event-data() -> ("NewVal"=w438:u32)  [unwired: 1 in, 5 out]
            n222 = call "getConfiguration.vi"("error in (no error)"=w431, "Xcite in"=w436) -> ("error out"=w430:errorcluster, "configuration"=w432:cluster{"intensities":u32[], "on_states":u8[]}, "Xcite out"=w433:refnum<class "Xcite.lvclass">)  [unwired: 7 in]
            n223 = in-place {
              in-place-border: w438 -> [w442]
              # "Convert to permille"
              n224 = in-place-cluster #10(w432) -> ("intensities"=w444:u32[])
              n225 = Replace Array Subset(array=w444, new element=w442, index=8) -> (w440:u32[])
              n226 = Multiply(x=w440, y=u32 10) -> (x*y=w439:u32[])
              n227 = in-place-cluster #10("intensities"=w439) -> (w437:cluster{"intensities":u32[], "on_states":u8[]})
            }
            n228 = call "setConfiguration.vi"("error in (no error)"=w430, "configuration"=w437, "Xcite in"=w433) -> ("error out"=w435:errorcluster, "Xcite out"=w434:refnum<class "Xcite.lvclass">)  [unwired: 7 in]
          }
          event "Channel1_On": Value Change {
            n229 = event-data() -> ("NewVal"=w454:bool)  [unwired: 1 in, 5 out]
            n230 = call "getConfiguration.vi"("error in (no error)"=w446, "Xcite in"=w452) -> ("error out"=w445:errorcluster, "configuration"=w448:cluster{"intensities":u32[], "on_states":u8[]}, "Xcite out"=w449:refnum<class "Xcite.lvclass">)  [unwired: 7 in]
            n231 = Boolean To (0,1)(Boolean=w454) -> (0, 1=w447:i16)
            n232 = in-place {
              in-place-border: w447 -> [w455]
              n233 = in-place-cluster #11(w448) -> ("on_states"=w458:u8[])
              n234 = Replace Array Subset(array=w458, new element=w455, index=0) -> (w457:u8[])
              n235 = in-place-cluster #11("on_states"=w457) -> (w453:cluster{"intensities":u32[], "on_states":u8[]})
            }
            n236 = call "setConfiguration.vi"("error in (no error)"=w445, "configuration"=w453, "Xcite in"=w449) -> ("error out"=w451:errorcluster, "Xcite out"=w450:refnum<class "Xcite.lvclass">)  [unwired: 7 in]
          }
          event "Channel2_On": Value Change {
            n237 = event-data() -> ("NewVal"=w468:bool)  [unwired: 1 in, 5 out]
            n238 = Boolean To (0,1)(Boolean=w468) -> (0, 1=w461:i16)
            n239 = call "getConfiguration.vi"("error in (no error)"=w460, "Xcite in"=w466) -> ("error out"=w459:errorcluster, "configuration"=w462:cluster{"intensities":u32[], "on_states":u8[]}, "Xcite out"=w463:refnum<class "Xcite.lvclass">)  [unwired: 7 in]
            n240 = in-place {
              in-place-border: w461 -> [w469]
              n241 = in-place-cluster #12(w462) -> ("on_states"=w472:u8[])
              n242 = Replace Array Subset(array=w472, new element=w469, index=1) -> (w471:u8[])
              n243 = in-place-cluster #12("on_states"=w471) -> (w467:cluster{"intensities":u32[], "on_states":u8[]})
            }
            n244 = call "setConfiguration.vi"("error in (no error)"=w459, "configuration"=w467, "Xcite in"=w463) -> ("error out"=w465:errorcluster, "Xcite out"=w464:refnum<class "Xcite.lvclass">)  [unwired: 7 in]
          }
          event "Channel3_On": Value Change {
            n245 = event-data() -> ("NewVal"=w482:bool)  [unwired: 1 in, 5 out]
            n246 = call "getConfiguration.vi"("error in (no error)"=w474, "Xcite in"=w480) -> ("error out"=w473:errorcluster, "configuration"=w476:cluster{"intensities":u32[], "on_states":u8[]}, "Xcite out"=w477:refnum<class "Xcite.lvclass">)  [unwired: 7 in]
            n247 = Boolean To (0,1)(Boolean=w482) -> (0, 1=w475:i16)
            n248 = in-place {
              in-place-border: w475 -> [w483]
              n249 = in-place-cluster #13(w476) -> ("on_states"=w486:u8[])
              n250 = Replace Array Subset(array=w486, new element=w483, index=2) -> (w485:u8[])
              n251 = in-place-cluster #13("on_states"=w485) -> (w481:cluster{"intensities":u32[], "on_states":u8[]})
            }
            n252 = call "setConfiguration.vi"("error in (no error)"=w473, "configuration"=w481, "Xcite in"=w477) -> ("error out"=w479:errorcluster, "Xcite out"=w478:refnum<class "Xcite.lvclass">)  [unwired: 7 in]
          }
          event "Channel4_On": Value Change {
            n253 = event-data() -> ("NewVal"=w496:bool)  [unwired: 1 in, 5 out]
            n254 = call "getConfiguration.vi"("error in (no error)"=w488, "Xcite in"=w494) -> ("error out"=w487:errorcluster, "configuration"=w490:cluster{"intensities":u32[], "on_states":u8[]}, "Xcite out"=w491:refnum<class "Xcite.lvclass">)  [unwired: 7 in]
            n255 = Boolean To (0,1)(Boolean=w496) -> (0, 1=w489:i16)
            n256 = in-place {
              in-place-border: w489 -> [w497]
              n257 = in-place-cluster #14(w490) -> ("on_states"=w500:u8[])
              n258 = Replace Array Subset(array=w500, new element=w497, index=3) -> (w499:u8[])
              n259 = in-place-cluster #14("on_states"=w499) -> (w495:cluster{"intensities":u32[], "on_states":u8[]})
            }
            n260 = call "setConfiguration.vi"("error in (no error)"=w487, "configuration"=w495, "Xcite in"=w491) -> ("error out"=w493:errorcluster, "Xcite out"=w492:refnum<class "Xcite.lvclass">)  [unwired: 7 in]
          }
          event "Channel5_On": Value Change {
            n261 = event-data() -> ("NewVal"=w510:bool)  [unwired: 1 in, 5 out]
            n262 = call "getConfiguration.vi"("error in (no error)"=w502, "Xcite in"=w508) -> ("error out"=w501:errorcluster, "configuration"=w504:cluster{"intensities":u32[], "on_states":u8[]}, "Xcite out"=w505:refnum<class "Xcite.lvclass">)  [unwired: 7 in]
            n263 = Boolean To (0,1)(Boolean=w510) -> (0, 1=w503:i16)
            n264 = in-place {
              in-place-border: w503 -> [w511]
              n265 = in-place-cluster #15(w504) -> ("on_states"=w514:u8[])
              n266 = Replace Array Subset(array=w514, new element=w511, index=4) -> (w513:u8[])
              n267 = in-place-cluster #15("on_states"=w513) -> (w509:cluster{"intensities":u32[], "on_states":u8[]})
            }
            n268 = call "setConfiguration.vi"("error in (no error)"=w501, "configuration"=w509, "Xcite in"=w505) -> ("error out"=w507:errorcluster, "Xcite out"=w506:refnum<class "Xcite.lvclass">)  [unwired: 7 in]
          }
          event "Channel6_On": Value Change {
            n269 = event-data() -> ("NewVal"=w524:bool)  [unwired: 1 in, 5 out]
            n270 = call "getConfiguration.vi"("error in (no error)"=w516, "Xcite in"=w522) -> ("error out"=w515:errorcluster, "configuration"=w518:cluster{"intensities":u32[], "on_states":u8[]}, "Xcite out"=w519:refnum<class "Xcite.lvclass">)  [unwired: 7 in]
            n271 = Boolean To (0,1)(Boolean=w524) -> (0, 1=w517:i16)
            n272 = in-place {
              in-place-border: w517 -> [w525]
              n273 = in-place-cluster #16(w518) -> ("on_states"=w528:u8[])
              n274 = Replace Array Subset(array=w528, new element=w525, index=5) -> (w527:u8[])
              n275 = in-place-cluster #16("on_states"=w527) -> (w523:cluster{"intensities":u32[], "on_states":u8[]})
            }
            n276 = call "setConfiguration.vi"("error in (no error)"=w515, "configuration"=w523, "Xcite in"=w519) -> ("error out"=w521:errorcluster, "Xcite out"=w520:refnum<class "Xcite.lvclass">)  [unwired: 7 in]
          }
          event "Channel7_On": Value Change {
            n277 = event-data() -> ("NewVal"=w538:bool)  [unwired: 1 in, 5 out]
            n278 = call "getConfiguration.vi"("error in (no error)"=w530, "Xcite in"=w536) -> ("error out"=w529:errorcluster, "configuration"=w532:cluster{"intensities":u32[], "on_states":u8[]}, "Xcite out"=w533:refnum<class "Xcite.lvclass">)  [unwired: 7 in]
            n279 = Boolean To (0,1)(Boolean=w538) -> (0, 1=w531:i16)
            n280 = in-place {
              in-place-border: w531 -> [w539]
              n281 = in-place-cluster #17(w532) -> ("on_states"=w542:u8[])
              n282 = Replace Array Subset(array=w542, new element=w539, index=6) -> (w541:u8[])
              n283 = in-place-cluster #17("on_states"=w541) -> (w537:cluster{"intensities":u32[], "on_states":u8[]})
            }
            n284 = call "setConfiguration.vi"("error in (no error)"=w529, "configuration"=w537, "Xcite in"=w533) -> ("error out"=w535:errorcluster, "Xcite out"=w534:refnum<class "Xcite.lvclass">)  [unwired: 7 in]
          }
          event "Channel8_On": Value Change {
            n285 = event-data() -> ("NewVal"=w552:bool)  [unwired: 1 in, 5 out]
            n286 = call "getConfiguration.vi"("error in (no error)"=w544, "Xcite in"=w550) -> ("error out"=w543:errorcluster, "configuration"=w546:cluster{"intensities":u32[], "on_states":u8[]}, "Xcite out"=w547:refnum<class "Xcite.lvclass">)  [unwired: 7 in]
            n287 = Boolean To (0,1)(Boolean=w552) -> (0, 1=w545:i16)
            n288 = in-place {
              in-place-border: w545 -> [w553]
              n289 = in-place-cluster #18(w546) -> ("on_states"=w556:u8[])
              n290 = Replace Array Subset(array=w556, new element=w553, index=7) -> (w555:u8[])
              n291 = in-place-cluster #18("on_states"=w555) -> (w551:cluster{"intensities":u32[], "on_states":u8[]})
            }
            n292 = call "setConfiguration.vi"("error in (no error)"=w543, "configuration"=w551, "Xcite in"=w547) -> ("error out"=w549:errorcluster, "Xcite out"=w548:refnum<class "Xcite.lvclass">)  [unwired: 7 in]
          }
          event "Channel9_On": Value Change {
            n293 = event-data() -> ("NewVal"=w566:bool)  [unwired: 1 in, 5 out]
            n294 = call "getConfiguration.vi"("error in (no error)"=w558, "Xcite in"=w564) -> ("error out"=w557:errorcluster, "configuration"=w560:cluster{"intensities":u32[], "on_states":u8[]}, "Xcite out"=w561:refnum<class "Xcite.lvclass">)  [unwired: 7 in]
            n295 = Boolean To (0,1)(Boolean=w566) -> (0, 1=w559:i16)
            n296 = in-place {
              in-place-border: w559 -> [w567]
              n297 = in-place-cluster #19(w560) -> ("on_states"=w570:u8[])
              n298 = Replace Array Subset(array=w570, new element=w567, index=8) -> (w569:u8[])
              n299 = in-place-cluster #19("on_states"=w569) -> (w565:cluster{"intensities":u32[], "on_states":u8[]})
            }
            n300 = call "setConfiguration.vi"("error in (no error)"=w557, "configuration"=w565, "Xcite in"=w561) -> ("error out"=w563:errorcluster, "Xcite out"=w562:refnum<class "Xcite.lvclass">)  [unwired: 7 in]
          }
        }
        n301 = call-dynamic "getRecordedImageCount.vi"("Camera in"=w299, "error in (no error)"=w298) -> ("Camera out"=w296:refnum<class "Camera.lvclass">, "recorded_image_count"=w286:u32, "error out"=w297:errorcluster)  [unwired: 11 in]
        "Recorded Images" <- w286
        n302 = Greater Than 0?(x=w286) -> (x > 0?=w287:bool)
        n303 = case shown="True" w287 {
          tunnel: [w571 w586] -> w300
          tunnel: w297 -> [w571 w583]
          tunnel: w296 -> [w572 w574]
          tunnel: [w572 w573] -> w295
          frame False {
          }
          frame True {
            # "U64"
            # "U32"
            # "U8"
            # "U16"
            # "Get latest image"
            n304 = local read "data_format"() -> (w575:T1)
            n305 = local read "Image"() -> (w580:T2)
            n306 = Bundle By Name(cluster=cluster{"x0":u64, "y0":u64, "x1":u64, "y1":u64} {"x0"=0, "y0"=0, "x1"=0, "y1"=0} ("roi"), "x0"="cropX0", "y0"="cropY0", "x1"="cropX1", "y1"="cropY1") -> (w587:cluster{"x0":u64, "y0":u64, "x1":u64, "y1":u64})
            n307 = local read "data_format"() -> (w582:T1)
            n308 = call-dynamic "image.vi"("Camera in"=w574, "data_format"=w582, "image_index"=u32 4294967295 ("dwImgIdx"), "crop"=w587, "error in (no error)"=w583) -> ("Camera out"=w573:refnum<class "Camera.lvclass">, "image (U8)"=w577:u8[][], "image (U32)"=w578:u32[][], "image (U64)"=w579:T13, "raw_image (U16)"=w576:u16[][], "error out"=w586:errorcluster)  [unwired: 2 in, 3 out]
            "rawImage" <- w576
            n309 = case shown="\"Mono8\"" w575 {
              tunnel: w580 -> [w594 w597 w600 w603 w606]
              tunnel: [w592 w595 w599 w601 w605] -> w581
              tunnel: w579 -> [_ _ _ w602 _]
              tunnel: w578 -> [_ _ w598 _ _]
              tunnel: w577 -> [_ w596 _ _ w604]
              tunnel: w576 -> [w593 _ _ _ _]
              frame "Mono16", Default {
                n310 = call "IMAQ ArrayToImage"("Image Pixels (U16)"=w593, "Image"=w594) -> ("Image Out"=w592:T2)  [unwired: 8 in, 1 out]
              }
              frame "Mono8" {
                n311 = call "IMAQ ArrayToImage"("Image Pixels (U8)"=w596, "Image"=w597) -> ("Image Out"=w595:T2)  [unwired: 8 in, 1 out]
              }
              frame "BGRA8", "RGBA8" {
                n312 = call "IMAQ ArrayToColorImage"("Image Pixels (U32)"=w598, "Image"=w600) -> ("Image Out"=w599:T2)  [unwired: 3 in, 1 out]
              }
              frame "BGRA16", "RGBA16" {
                n313 = call "IMAQ ArrayToColorImage"("Image"=w603, "Image Pixels (U64)"=w602) -> ("Image Out"=w601:T2)  [unwired: 3 in, 1 out]
              }
              frame "CompressedMono8" {
                n314 = call "IMAQ ArrayToImage"("Image Pixels (U8)"=w604, "Image"=w606) -> ("Image Out"=w605:T2)  [unwired: 8 in, 1 out]
              }
            }
            n315 = local write "Image"(w581) -> ()
          }
        }
        n316 = Or(x="Stop Record", y="Quit") -> (x .or. y?=w305:bool)
        n317 = case shown="True" w305 {
          tunnel: w300 -> [w617 w618]
          tunnel: [w616 w620] -> w289
          tunnel: [w617 w621] -> w288
          tunnel: w295 -> [w616 w619]
          frame False {
          }
          frame True {
            n318 = call-dynamic "stop.vi"("error in (no error)"=w618, "Camera in"=w619) -> ("error out"=w621:errorcluster, "Camera out"=w620:refnum<class "Camera.lvclass">)  [unwired: 8 in]
          }
        }
        n319 = Unbundle By Name(w288) -> ("status"=w303:bool)
        n320 = Not(x=w302) -> (.not. x?=w301:bool)
        n321 = Or(x=w301, y=w303) -> (x .or. y?=w304:bool)
      }
      n322 = property on="Quit" class="Bool (strict)"("DisabledEnum"=T4."Enabled" ("Disabled")) -> ()  [unwired: 2 in, 2 out]
    }
    frame #6 {
      w626 = FALSE ("Channel1_On")
      w627 = T4."Disabled" ("Disabled")
      # "Switch off all X-Cite channels"
      # "Update image index"
      # "Reset Stop Record button"
      # "Get Status, e.g recorded image count"
      n323 = local read "dwImgCount"() -> (w636:u32)
      n324 = call-dynamic "getRecordedImageCount.vi"("Camera in"=w630, "error in (no error)"=w637) -> ("Camera out"=w629:refnum<class "Camera.lvclass">, "recorded_image_count"=w628:u32, "error out"=w635:errorcluster)  [unwired: 11 in]
      n325 = local write "Channel1_On"(w626) -> ()
      n326 = local write "Channel2_On"(w626) -> ()
      n327 = local write "Channel3_On"(w626) -> ()
      n328 = local write "Channel4_On"(w626) -> ()
      n329 = local write "Channel5_On"(w626) -> ()
      n330 = local write "Channel6_On"(w626) -> ()
      n331 = local write "Channel7_On"(w626) -> ()
      n332 = local write "Channel8_On"(w626) -> ()
      n333 = local write "Channel9_On"(w626) -> ()
      n334 = call "switchOff.vi"("error in (no error)"=w624, "Xcite in"=w625) -> ("error out"=w622:errorcluster, "Xcite out"=w623:refnum<class "Xcite.lvclass">)  [unwired: 8 in]
      n335 = local write "Recorded Images"(w628) -> ()
      n336 = Max & Min(x=w628, y=w636) -> (min(x,y)=w638:u32)  [unwired: 1 out]
      n337 = Decrement(x=w638) -> (x-1=w633:u32)
      n338 = local write "Stop Record"(FALSE ("Stop Record")) -> ()
      n339 = property on="Stop Record" class="Bool (strict)"("DisabledEnum"=T4."Disabled and Grayed Out" ("Disabled")) -> ()  [unwired: 2 in, 2 out]
      n340 = property on="Image Index" class="DigNum (strict)"("DisabledEnum"=T4."Enabled" ("Disabled")) -> ()  [unwired: 2 in, 2 out]
      n341 = property on="Channel1_On" class="Bool (strict)"("DisabledEnum"=w627) -> ()  [unwired: 2 in, 2 out]
      n342 = property on="Channel2_On" class="Bool (strict)"("DisabledEnum"=w627) -> ()  [unwired: 2 in, 2 out]
      n343 = property on="Channel3_On" class="Bool (strict)"("DisabledEnum"=w627) -> ()  [unwired: 2 in, 2 out]
      n344 = property on="Channel4_On" class="Bool (strict)"("DisabledEnum"=w627) -> ()  [unwired: 2 in, 2 out]
      n345 = property on="Channel5_On" class="Bool (strict)"("DisabledEnum"=w627) -> ()  [unwired: 2 in, 2 out]
      n346 = property on="Channel6_On" class="Bool (strict)"("DisabledEnum"=w627) -> ()  [unwired: 2 in, 2 out]
      n347 = property on="Channel7_On" class="Bool (strict)"("DisabledEnum"=w627) -> ()  [unwired: 2 in, 2 out]
      n348 = property on="Channel8_On" class="Bool (strict)"("DisabledEnum"=w627) -> ()  [unwired: 2 in, 2 out]
      n349 = property on="Channel9_On" class="Bool (strict)"("DisabledEnum"=w627) -> ()  [unwired: 2 in, 2 out]
      n350 = property on="Trigger" class="Bool (strict)"("DisabledEnum"=T4."Disabled and Grayed Out" ("Disabled"), "Value"=FALSE ("Trigger")) -> ()  [unwired: 2 in, 2 out]
      n351 = property on="Image Index" class="DigNum (strict)"("Maximum"=w633) -> ()  [unwired: 2 in, 2 out]
    }
    frame #7 {
      # "Do the image readout"
      n352 = Greater Than 0?(x=w643) -> (x > 0?=w644:bool)
      n353 = case shown="True" w644 {
        tunnel: w648 -> [w649 w654]
        tunnel: [w649 w653] -> w647
        tunnel: w646 -> [w650 w652]
        tunnel: [w650 w651] -> w645
        frame False {
        }
        frame True {
          n354 = while {
            shift-right: [w668] -> w653
            shift-left: w654 -> [w676]
            shift-right: [w655] -> w651
            shift-left: w652 -> [w656]
            stop <- w670 stop-if-true
            n355 = local read "cropX0"() -> (w666:u64)
            n356 = local read "cropY0"() -> (w667:u64)
            n357 = local read "cropX1"() -> (w674:u64)
            n358 = local read "cropY1"() -> (w673:u64)
            n359 = local read "data_format"() -> (w664:T1)
            n360 = Bundle By Name(cluster=cluster{"x0":u64, "y0":u64, "x1":u64, "y1":u64} {"x0"=0, "y0"=0, "x1"=0, "y1"=0} ("roi"), "x0"=w666, "y0"=w667, "x1"=w674, "y1"=w673) -> (w675:cluster{"x0":u64, "y0":u64, "x1":u64, "y1":u64})
            n361 = local read "data_format"() -> (w657:T1)
            n362 = call-dynamic "image.vi"("Camera in"=w656, "data_format"=w664, "image_index"="Image Index", "crop"=w675, "error in (no error)"=w676) -> ("Camera out"=w655:refnum<class "Camera.lvclass">, "image (U8)"=w660:u8[][], "image (U32)"=w659:u32[][], "image (U64)"=w658:T13, "raw_image (U16)"=w661:u16[][], "error out"=w668:errorcluster)  [unwired: 2 in, 3 out]
            n363 = local read "Image"() -> (w662:T2)
            n364 = case shown="\"Mono8\"" w657 {
              tunnel: w662 -> [w679 w682 w685 w688 w691]
              tunnel: [w677 w680 w684 w686 w690] -> w663
              tunnel: w658 -> [_ _ _ w687 _]
              tunnel: w659 -> [_ _ w683 _ _]
              tunnel: w660 -> [_ w681 _ _ w689]
              tunnel: w661 -> [w678 _ _ _ _]
              frame "Mono16", Default {
                n365 = call "IMAQ ArrayToImage"("Image Pixels (U16)"=w678, "Image"=w679) -> ("Image Out"=w677:T2)  [unwired: 8 in, 1 out]
              }
              frame "Mono8" {
                n366 = call "IMAQ ArrayToImage"("Image Pixels (U8)"=w681, "Image"=w682) -> ("Image Out"=w680:T2)  [unwired: 8 in, 1 out]
              }
              frame "BGRA8", "RGBA8" {
                n367 = call "IMAQ ArrayToColorImage"("Image Pixels (U32)"=w683, "Image"=w685) -> ("Image Out"=w684:T2)  [unwired: 3 in, 1 out]
              }
              frame "BGRA16", "RGBA16" {
                n368 = call "IMAQ ArrayToColorImage"("Image"=w688, "Image Pixels (U64)"=w687) -> ("Image Out"=w686:T2)  [unwired: 3 in, 1 out]
              }
              frame "CompressedMono8" {
                n369 = call "IMAQ ArrayToImage"("Image Pixels (U8)"=w689, "Image"=w691) -> ("Image Out"=w690:T2)  [unwired: 8 in, 1 out]
              }
            }
            n370 = local write "rawImage"(w661) -> ()
            n371 = Unbundle By Name(w668) -> ("status"=w671:bool)
            n372 = local read "Quit"() -> (w672:bool)
            n373 = local write "Image"(w663) -> ()
            n374 = Or(x=w671, y=w672) -> (x .or. y?=w670:bool)
          }
        }
      }
    }
    frame #8 {
      # "Close connection to X-Cite"
      # "Delete image"
      # "Close everything"
      # "Reset Quit button"
      n375 = local read "Image"() -> (w694:T2)
      n376 = call "close.vi"("error in (no error)"=w692, "Xcite in"=w693) -> ()  [unwired: 9 in, 1 out]
      n377 = call-dynamic "close.vi"("error in (no error)"=w697, "Camera in"=w695) -> ("error out"=→"Error":errorcluster)  [unwired: 9 in]
      n378 = call "IMAQ Dispose"("Image"=w694) -> ()  [unwired: 5 in, 1 out]
      n379 = local write "Quit"(FALSE ("Stop Record")) -> ()
    }
  }
  n380 = while {
    stop <- w699 stop-if-true
    # "Event structure for parameter checking"
    n381 = event shown="[4] \"cropX0\": Value Change" {
      selector: _ -> [_ _ _ _ _ _ _ _ _]
      dyn-events: _ -> [_ _ _ _ _ _ _ _ _]
      timeout: 1000 -> [_ _ _ _ _ _ _ _ _]
      tunnel: [_ TRUE _ _ _ _ _ _ _] -> w699
      event Timeout {
        n382 = event-data() -> ()  [unwired: 1 in, 3 out]
      }
      event "Quit": Value Change {
        n383 = event-data() -> ()  [unwired: 1 in, 6 out]
      }
      event "Image Width": Value Change {
        n384 = event-data() -> ("NewVal"=w702:u64)  [unwired: 1 in, 5 out]
        n385 = Decrement(x=w702) -> (x-1=w703:u64)
        n386 = property on="cropX0" class="DigNum (strict)"("Maximum"=w703) -> ()  [unwired: 2 in, 2 out]
        n387 = property on="cropX1" class="DigNum (strict)"("Maximum"=w702) -> ()  [unwired: 2 in, 2 out]
      }
      event "Image Height": Value Change {
        n388 = event-data() -> ("NewVal"=w704:u64)  [unwired: 1 in, 5 out]
        n389 = Decrement(x=w704) -> (x-1=w705:u64)
        n390 = property on="cropY1" class="DigNum (strict)"("Maximum"=w704) -> ()  [unwired: 2 in, 2 out]
        n391 = property on="cropY0" class="DigNum (strict)"("Maximum"=w705) -> ()  [unwired: 2 in, 2 out]
      }
      event "cropX0": Value Change {
        n392 = event-data() -> ("NewVal"=w706:u64)  [unwired: 1 in, 5 out]
        n393 = local read "cropX1"() -> (w708:u64)
        n394 = Greater Or Equal?(x=w706, y=w708) -> (x >= y?=w707:bool)
        n395 = case shown="True" w707 {
          tunnel: w706 -> [_ w710]
          frame False {
          }
          frame True {
            n396 = Increment(x=w710) -> (x+1=w709:u64)
            n397 = local write "cropX1"(w709) -> ()
          }
        }
      }
      event Panel Close? {
        n398 = event-data() -> ()  [unwired: 1 in, 4 out]
        n399 = One Button Dialog(message="Please click on \"Quit Application\"\nbutton before closing!") -> (true=w711:bool)  [unwired: 1 in]
        n400 = event-data("Discard?"=w711) -> ()  [unwired: 1 in, 1 out]
      }
      event "cropY0": Value Change {
        n401 = event-data() -> ("NewVal"=w713:u64)  [unwired: 1 in, 5 out]
        n402 = local read "cropY1"() -> (w715:u64)
        n403 = Greater Or Equal?(x=w713, y=w715) -> (x >= y?=w714:bool)
        n404 = case shown="True" w714 {
          tunnel: w713 -> [_ w717]
          frame False {
          }
          frame True {
            n405 = Increment(x=w717) -> (x+1=w716:u64)
            n406 = local write "cropY1"(w716) -> ()
          }
        }
      }
      event "cropX1": Value Change {
        n407 = event-data() -> ("NewVal"=w718:u64)  [unwired: 1 in, 5 out]
        n408 = local read "cropX0"() -> (w720:u64)
        n409 = Less Or Equal?(x=w718, y=w720) -> (x <= y?=w719:bool)
        n410 = case shown="False" w719 {
          tunnel: w718 -> [_ w722]
          frame False {
          }
          frame True {
            n411 = Decrement(x=w722) -> (x-1=w721:u64)
            n412 = local write "cropX0"(w721) -> ()
          }
        }
      }
      event "cropY1": Value Change {
        n413 = event-data() -> ("NewVal"=w723:u64)  [unwired: 1 in, 5 out]
        n414 = local read "cropY0"() -> (w725:u64)
        n415 = Less Or Equal?(x=w723, y=w725) -> (x <= y?=w724:bool)
        n416 = case shown="True" w724 {
          tunnel: w723 -> [_ w727]
          frame False {
          }
          frame True {
            n417 = Decrement(x=w727) -> (x-1=w726:u64)
            n418 = local write "cropY0"(w726) -> ()
          }
        }
      }
    }
  }
